vi "myRIO_BRig_RT_dataMTrig_Audio_N__L.vi"() -> (2 "output_Audio_N__L":i32)   [LabVIEW 2014]
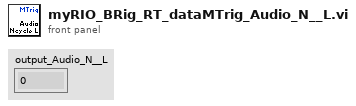
[diagram p1: front panel]
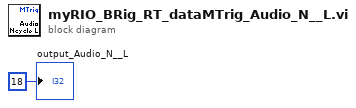
[diagram p0: block diagram]
diagram:
  "output_Audio_N__L" <- 18 ("output_iBlock")
